vi "ook_sync.vi"() -> ()   [LabVIEW 2009]
uses:
  <vilib>/Analysis/NI_AALBase.lvlib
panel:
  in  "位相":dbl
  in  "Q":dbl
  in  "雑音振幅":dbl
  out "誤り率":dbl
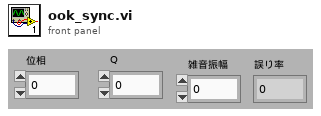
[diagram p1: front panel]
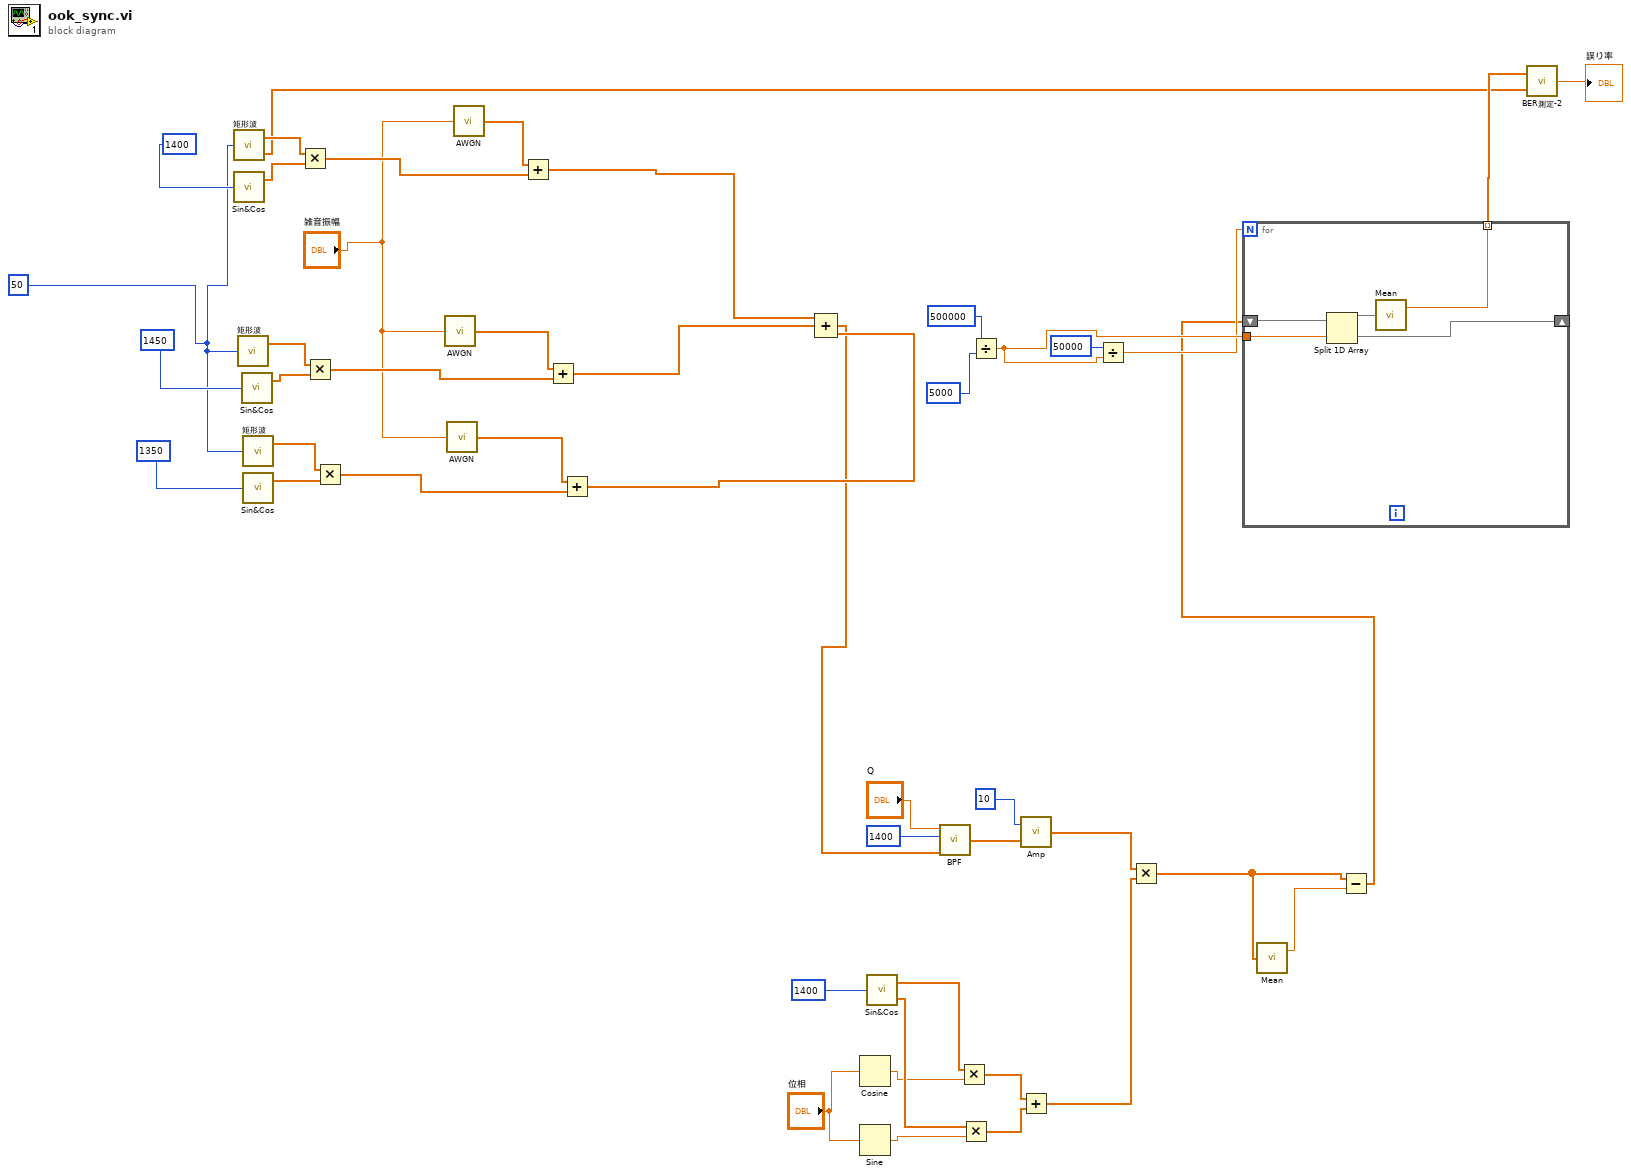
[diagram p0: block diagram]
diagram:
  w31 = 50
  n1 = call "矩形波.vi"("信号周波数 [kHz]"=w31) -> ("矩形波"=w41:dbl[], "送信データ"=w23:dbl[])
  n2 = call "Sin&Cos.vi"("周波数[kHz]"=1400) -> ("sin"=w42:dbl[])  [unwired: 1 out]
  n3 = call "矩形波.vi"("信号周波数 [kHz]"=w31) -> ("矩形波"=w44:dbl[])  [unwired: 1 out]
  n4 = call "Sin&Cos.vi"("周波数[kHz]"=1450) -> ("sin"=w43:dbl[])  [unwired: 1 out]
  n5 = call "矩形波.vi"("信号周波数 [kHz]"=w31) -> ("矩形波"=w45:dbl[])  [unwired: 1 out]
  n6 = call "Sin&Cos.vi"("周波数[kHz]"=1350) -> ("sin"=w46:dbl[])  [unwired: 1 out]
  n7 = Multiply(x=w41, y=w42) -> (x*y=w26:dbl[])
  n8 = Multiply(x=w44, y=w43) -> (x*y=w35:dbl[])
  n9 = Multiply(x=w45, y=w46) -> (x*y=w33:dbl[])
  n10 = call "AWGN.vi"("振幅値"="雑音振幅") -> ("出力"=w36:dbl[])
  n11 = call "AWGN.vi"("振幅値"="雑音振幅") -> ("出力"=w34:dbl[])
  n12 = call "AWGN.vi"("振幅値"="雑音振幅") -> ("出力"=w37:dbl[])
  n13 = Add(x=w37, y=w26) -> (x+y=w22:dbl[])
  n14 = Add(x=w36, y=w35) -> (x+y=w21:dbl[])
  n15 = Add(x=w34, y=w33) -> (x+y=w20:dbl[])
  n16 = Compound Arithmetic op=ADD(w22, w21, w20) -> (w3:dbl[])
  n17 = Cosine(x="位相") -> (cos(x)=w6:dbl)
  n18 = Sine(x="位相") -> (sin(x)=w4:dbl)
  n19 = call "Sin&Cos.vi"("周波数[kHz]"=1400) -> ("sin"=w12:dbl[], "cos"=w11:dbl[])
  n20 = call "BPF.vi"("X"=w3, "中心周波数 [kHz]"=1400, "Q"="Q") -> ("BPF出力"=w17:dbl[])  [unwired: 1 in]
  n21 = Multiply(x=w12, y=w6) -> (x*y=w10:dbl[])
  n22 = Multiply(x=w11, y=w4) -> (x*y=w9:dbl[])
  n23 = Divide(x=500000, y=5000) -> (x/y=w29:dbl)
  n24 = call "Amp.vi"("入力"=w17, "増幅率"=10) -> ("出力"=w14:dbl[])
  n25 = Add(x=w10, y=w9) -> (x+y=w8:dbl[])
  n26 = Divide(x=50000, y=w29) -> (x/y=w28:dbl)
  n27 = Multiply(x=w14, y=w8) -> (x*y=w1:dbl[])
  n28 = call <vilib>:"Mean.vi"("X"=w1) -> ("mean"=w7:dbl)  [unwired: 1 out]
  n29 = Subtract(x=w1, y=w7) -> (x-y=w2:dbl[])
  n30 = for {
    N: w28 -> [_]
    shift-right: [w48] -> _
    shift-left: w2 -> [w51]
    tunnel: [w49] -> w27 mode=indexing
    tunnel: w29 -> [w47]
    n31 = Split 1D Array(array=w51, index=w47) -> (first subarray=w50:dbl[], second subarray=w48:dbl[])
    n32 = call <vilib>:"Mean.vi"("X"=w50) -> ("mean"=w49:dbl)  [unwired: 1 out]
  }
  n33 = call "BER測定-2.vi"("参照データ"=w23, "入力データ"=w27) -> ("BER"=→"誤り率":dbl)
